vi "DSF.Engine.Interface.Transceiver.New.vi"(5 "FIFO Debug Flags":refnum<class "DSF.Engine.Debug Flags.FIFO.lvclass">, 7 "fifo depths (10)":u32=10, 8 "error in (no error)":errorcluster, 10 "error size (512 B)":T1=enum."512-byte", 11 "Transceiver Interface type":refnum<class "DSF.Engine.Interface.Transceiver.lvclass">) -> (0 "error out":errorcluster, 3 "Transceiver Interface":refnum<class "DSF.Engine.Interface.Transceiver.lvclass">)   [LabVIEW 2017, in "DSF.Engine.lvlib" / "DSF.Engine.Interface.Transceiver.lvclass"]
uses:
  DSF.Engine.Interface.Transceiver.lvclass
  C:/Git/DSF/Source/Engine/Classes/Interface/DSF.Engine.Interface.lvclass
  DSF.Engine.Interface.Error Queue.Sizes.ctl
  Debug/DSF.Engine.Debug Flags.FIFO.lvclass
  DSF.Engine.Interface.lvclass
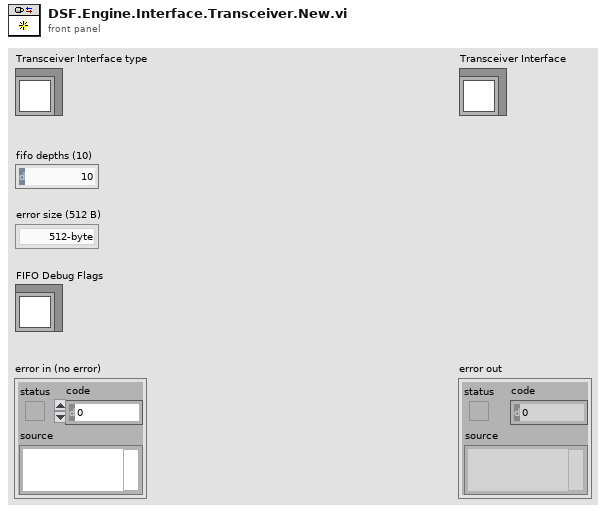
[diagram p1: front panel]
types:
  T1 = typedef "DSF.Engine.lvlib/DSF.Engine.Interface.lvclass/DSF.Engine.Interface.Error Queue.Sizes.ctl" = enum16{"256-byte", "512-byte", "1024-byte"}
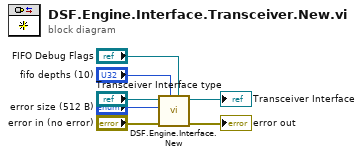
[diagram p0: block diagram]
diagram:
  n1 = call "DSF.Engine.Interface.New.vi"("FIFO Debug Flags"="FIFO Debug Flags", "fifo/queue depths (10)"="fifo depths (10)", "error in (no error)"="error in (no error)", "error size (512 B)"="error size (512 B)", "Interface type"="Transceiver Interface type") -> ("error out"=→"error out":errorcluster, "Interface"=→"Transceiver Interface":refnum<class "DSF.Engine.Interface.Transceiver.lvclass">)  [unwired: 5 in]
